vi "OPCWrite.vi"() -> ()   [LabVIEW 2021]
panel:
  out "Waveform Chart":dbl(graph)
  in  "SFilter Enabled":bool
  in  "stop":bool
  out "Temperature":dbl
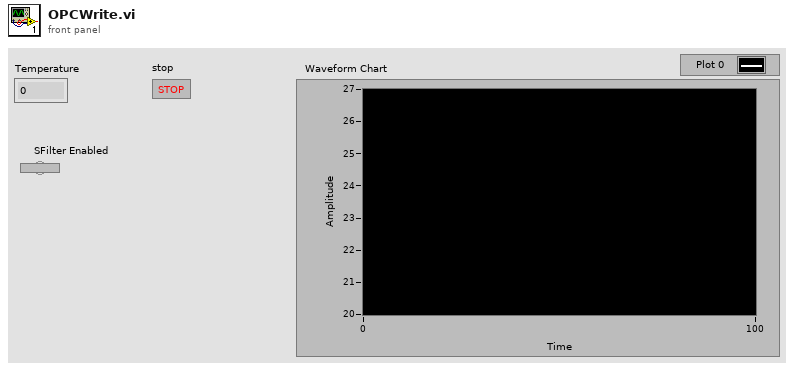
[diagram p1: front panel]
types:
  T1 = enum16{"Read", "Write", "ReadWrite", "BufferedRead", "BufferedReadWrite"}
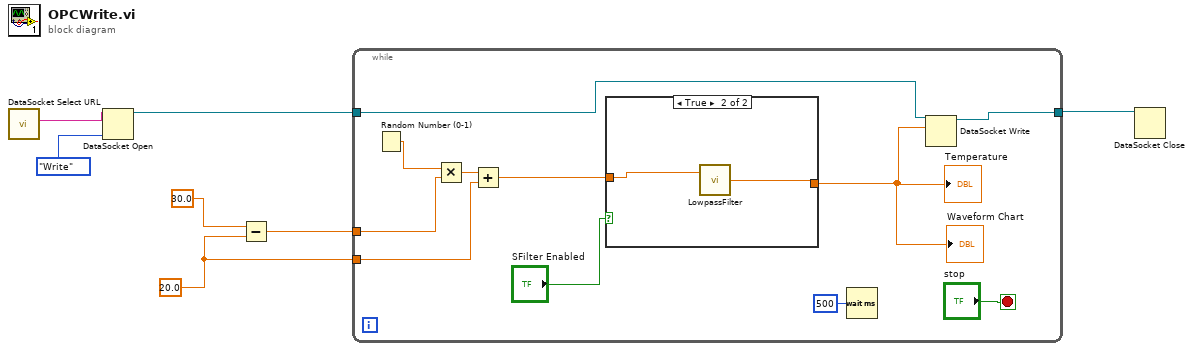
[diagram p0: block diagram]
diagram:
  w3 = 20.0
  n1 = call <vilib>:"DataSocket Select URL.vi"() -> ("URL"=w7:string)  [unwired: 9 in, 2 out]
  n2 = DataSocket Open(10:T1."Write" ("mode"), 11:w7) -> (3:w2:refnum<k13>)  [unwired: 2 in, 1 out]
  n3 = Subtract(x=30.0, y=w3) -> (x-y=w4:dbl)
  n4 = while {
    tunnel: w4 -> [w17]
    tunnel: w3 -> [w16]
    tunnel: w2 -> [w11]
    tunnel: [w12] -> w1
    stop <- "stop" stop-if-true
    n5 = Random Number (0-1)() -> (number: 0 to 1=w18:dbl)
    n6 = Multiply(x=w18, y=w17) -> (x*y=w15:dbl)
    n7 = Add(x=w15, y=w16) -> (x+y=w10:dbl)
    n8 = case shown="True" "SFilter Enabled" {
      tunnel: [w19 w21] -> w8
      tunnel: w10 -> [w19 w20]
      frame False {
      }
      frame True {
        n9 = call "LowpassFilter.vi"("Y(n)"=w20) -> ("Y(n+1)"=w21:dbl)  [unwired: 2 in]
      }
    }
    "Temperature" <- w8
    "Waveform Chart" <- w8
    n10 = Wait (ms)(milliseconds to wait=u32 500) -> ()  [unwired: 1 out]
    n11 = DataSocket Write(10:w8, 11:w11) -> (3:w12:refnum<k13>)  [unwired: 2 in, 2 out]
  }
  n12 = DataSocket Close(11:w1) -> ()  [unwired: 2 in, 2 out]
